vi "Configure Voltage Input Connection.vi"(8 "error in (no error)":errorcluster, 10 "Enable Guard (F: Disable)":bool, 11 "VISA resource name":refnum<visa-resource-name>) -> (0 "error out":errorcluster, 3 "VISA resource name out":refnum<visa-resource-name>)   [LabVIEW 2019, in "Keithley 6517.lvlib"]
doc: "Configures the voltage input terminal connection.\n\nNote:\nVoltage measurement should be enabled from <b>Configure Measurement Function.vi</b>."
uses:
  Keithley 6517.lvlib
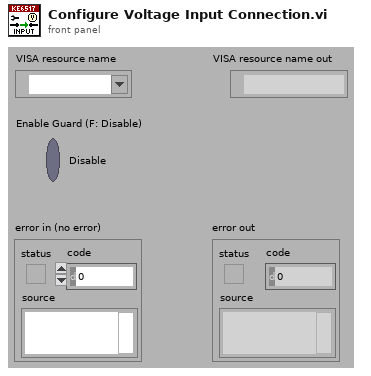
[diagram p1: front panel]
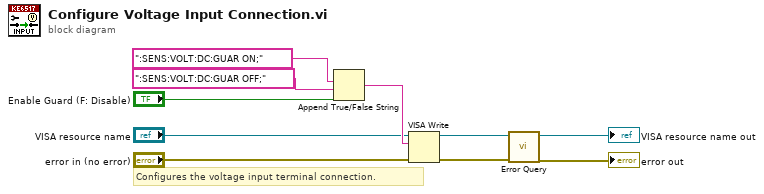
[diagram p0: block diagram]
diagram:
  # "Configures the voltage input terminal connection."
  n1 = Append True/False String(1:"Enable Guard (F: Disable)", 2:":SENS:VOLT:DC:GUAR OFF;", 3:":SENS:VOLT:DC:GUAR ON;") -> (0:w7:string)  [unwired: 1 in]
  n2 = VISA Write(VISA resource name="VISA resource name", write buffer=w7, error in (no error)="error in (no error)") -> (VISA resource name out=w4:refnum<visa-resource-name>, error out=w3:errorcluster)  [unwired: 1 out]
  n3 = call "Error Query.vi"("error in (no error)"=w3, "VISA resource name"=w4) -> ("error out"=→"error out":errorcluster, "VISA resource name out"=→"VISA resource name out":refnum<visa-resource-name>)  [unwired: 6 in, 2 out]
